vi "ref Periodic Tasks.vi"(8 "error in":errorcluster) -> ()   [LabVIEW 2020]
doc: "This VI runs in parallel to other tasks. It can contain as many user-defined periodic loops as you need. These can carry out PID or other sorts of timed response."
uses:
  <vilib>/Rock Robotics/Network Tables/NT Write Number.vi
  <vilib>/Rock Robotics/Network Tables/NT Write String.vi
  <vilib>/Rock Robotics/WPI/ThirdParty/Sensors/navX/_TypeDefs/FRIC_navX_DeviceNumbersTypeDef.ctl
  <vilib>/Rock Robotics/SystemInterfaces/i2clib/i2c_bus.ctl
  <vilib>/Rock Robotics/WPI/ThirdParty/Sensors/navX/_Processing Loop/FRIC_navX_Internal_I2C_ProcessingLoop.vi
  <vilib>/Rock Robotics/Network Tables/NT Read Number.vi
  <vilib>/Rock Robotics/WPI/Ultrasonic/WPI_SonarSRF04DigitalGetRange.vi
  <vilib>/Rock Robotics/WPI/Ultrasonic/WPI_SonarSRF04DigitalRefNum Registry Get.vi
  <vilib>/Rock Robotics/WPI/Ultrasonic/WPI_UltrasonicRangeUnits.ctl
  <vilib>/Rock Robotics/SystemInterfaces/DIO/FPGA_DIOPWMChannel.ctl
  <vilib>/Rock Robotics/WPI/PWM/WPI_PWMDeadband.ctl
  <vilib>/Rock Robotics/WPI/PWM/Servo/WPI_ServoDeviceRef.ctl
panel:
  in  "SONAR ref names":string[](array[string])=["BALL1", "BALL2"]
  in  "Cluster":T4={"RefAngle"="", "RefSetAngle"="", "ServoDeviceRef"={"DeviceStatus"={"status"=FALSE, "code"=0, "source"=""}, "PWM Channel"=enum."Invalid", "DeadBand"={"Name"="", "maxPositivePwm"=0, "minPositivePwm"=0, "centerPwm"=0, "maxNegativePwm"=0, "minNegativePwm"=0, "angularRange"=0}}}
  in  "list of NEO RefNum":string[](array[string])=["ARMLEFT", "ARMRIGHT"]
  in  "list of Falcon 500 RefNum":string[](array[string])=["DriveLEFT", "DriveRIGHT", "ClimberLEFT", "ClimberRIGHT", "SHOOTER"]
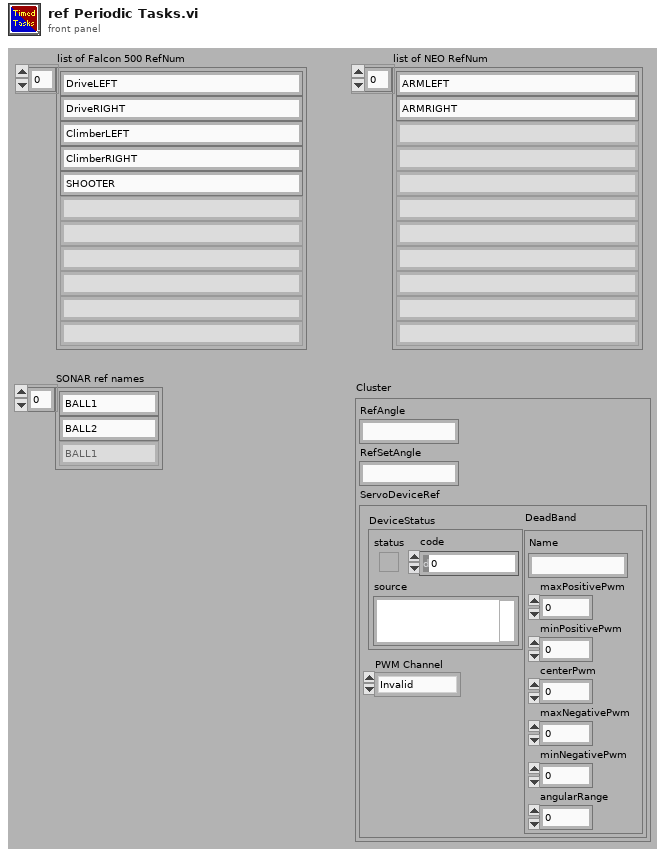
[diagram p1: front panel]
types:
  T1 = typedef "WPI_ServoDeviceRef.ctl" = cluster{"DeviceStatus":errorcluster, "PWM Channel":T2, "DeadBand":T3}
  T2 = typedef "FPGA_DIOPWMChannel.ctl" = enum8{"PWM 0", "PWM 1", "PWM 2", "PWM 3", "PWM 4", "PWM 5", "PWM 6", "PWM 7", "PWM 8", "PWM 9", "PWM MXP 0", "PWM MXP 1", "PWM MXP 2", "PWM MXP 3", "PWM MXP 4", "PWM MXP 5", "PWM MXP 6", "PWM MXP 7", "PWM MXP 8", "PWM MXP 9", "Invalid"}
  T3 = typedef "WPI_PWMDeadband.ctl" = cluster{"Name":string, "maxPositivePwm":i32, "minPositivePwm":i32, "centerPwm":i32, "maxNegativePwm":i32, "minNegativePwm":i32, "angularRange":u16}
  T4 = cluster{"RefAngle":string, "RefSetAngle":string, "ServoDeviceRef":T1}
  T5 = cluster{"RefAngle":string, "RefSetAngle":string, "ServoDeviceRef":T1}[]
  T6 = typedef "i2c_bus.ctl" = enum16{"I2C On-Board", "I2C MXP", "Invalid"}
  T7 = typedef "FRIC_navX_DeviceNumbersTypeDef.ctl" = enum16{"Dev0", "Dev1", "Dev2", "Dev3"}
  T8 = typedef "WPI_UltrasonicDeviceRef.ctl" = cluster{"DevStatus":errorcluster, "Ping Channel":T9, "Echo Channel":T9, "CntIndex":T10}
  T9 = typedef "FPGA_DIOChannel.ctl" = enum8{"DIO 0", "DIO 1", "DIO 2", "DIO 3", "DIO 4", "DIO 5", "DIO 6", "DIO 7", "DIO 8", "DIO 9", "DIO MXP 0", "DIO MXP 1", "DIO MXP 2", "DIO MXP 3", "DIO MXP 4", "DIO MXP 5", "DIO MXP 6", "DIO MXP 7", "DIO MXP 8", "DIO MXP 9", "DIO MXP 10", "DIO MXP 11", "DIO MXP 12", "DIO MXP 13", "DIO MXP 14", "DIO MXP 15", "SPI Port CS1", "SPI Port CS2", "SPI Port CS3", "SPI Port MISO", "SPI Port MOSI", "Invalid"}
  T10 = typedef "FPGA_CounterCtrSystemIndex.ctl" = enum8{"Ctr 0", "Ctr 1", "Ctr 2", "Ctr 3", "Ctr 4", "Ctr 5", "Ctr 6", "Ctr 7", "Invalid"}
  T11 = typedef "WPI_JoystickDevRef.ctl" = cluster{"Device":T12}
  T12 = typedef "WPI_JoystickDeviceEnum.ctl" = enum16{"USB 0", "USB 1", "USB 2", "USB 3", "USB 4", "USB 5"}
  T13 = typedef "WPI_RobotDriveDevRef.ctl" = cluster{"DevStatus":errorcluster, "Motors[]":T14[], "Square Inputs":bool, "Max Output":dbl}
  T14 = typedef "WPI_MotorControlDeviceRef.ctl" = cluster{"DeviceStatus":errorcluster, "Type":T15, "PWM":cluster{"PWM Channel":T2, "DeadBand":T3}, "CAN":cluster{"Device Number":u8, "SetOutput VI Ref":variant, "GetOutput VI Ref":variant, "Enable VI Ref":variant, "Disable VI Ref":variant, "Data":variant}, "Invert":bool, "DIO PWM":cluster{"PWM \"Enable\" Channel":T2, "DIOChannel":T9, "PWM Rate":dbl}}
  T15 = typedef "WPI_MotorControlType.ctl" = enum16{"PWM", "CAN", "DIO PWM"}
  T16 = cluster{"JoystickDevRef":T11, "RobotDriveDevRef":T13}
  T17 = typedef "WPI_UltrasonicRangeUnits.ctl" = enum16{"inches", "mm"}
  T18 = typedef "WPI_DriverStationPositionInfo.ctl" = enum16{"1", "2", "3"}
  T19 = typedef "WPI_DriverStationAllianceInfo.ctl" = enum16{"Red", "Blue", "Invalid"}
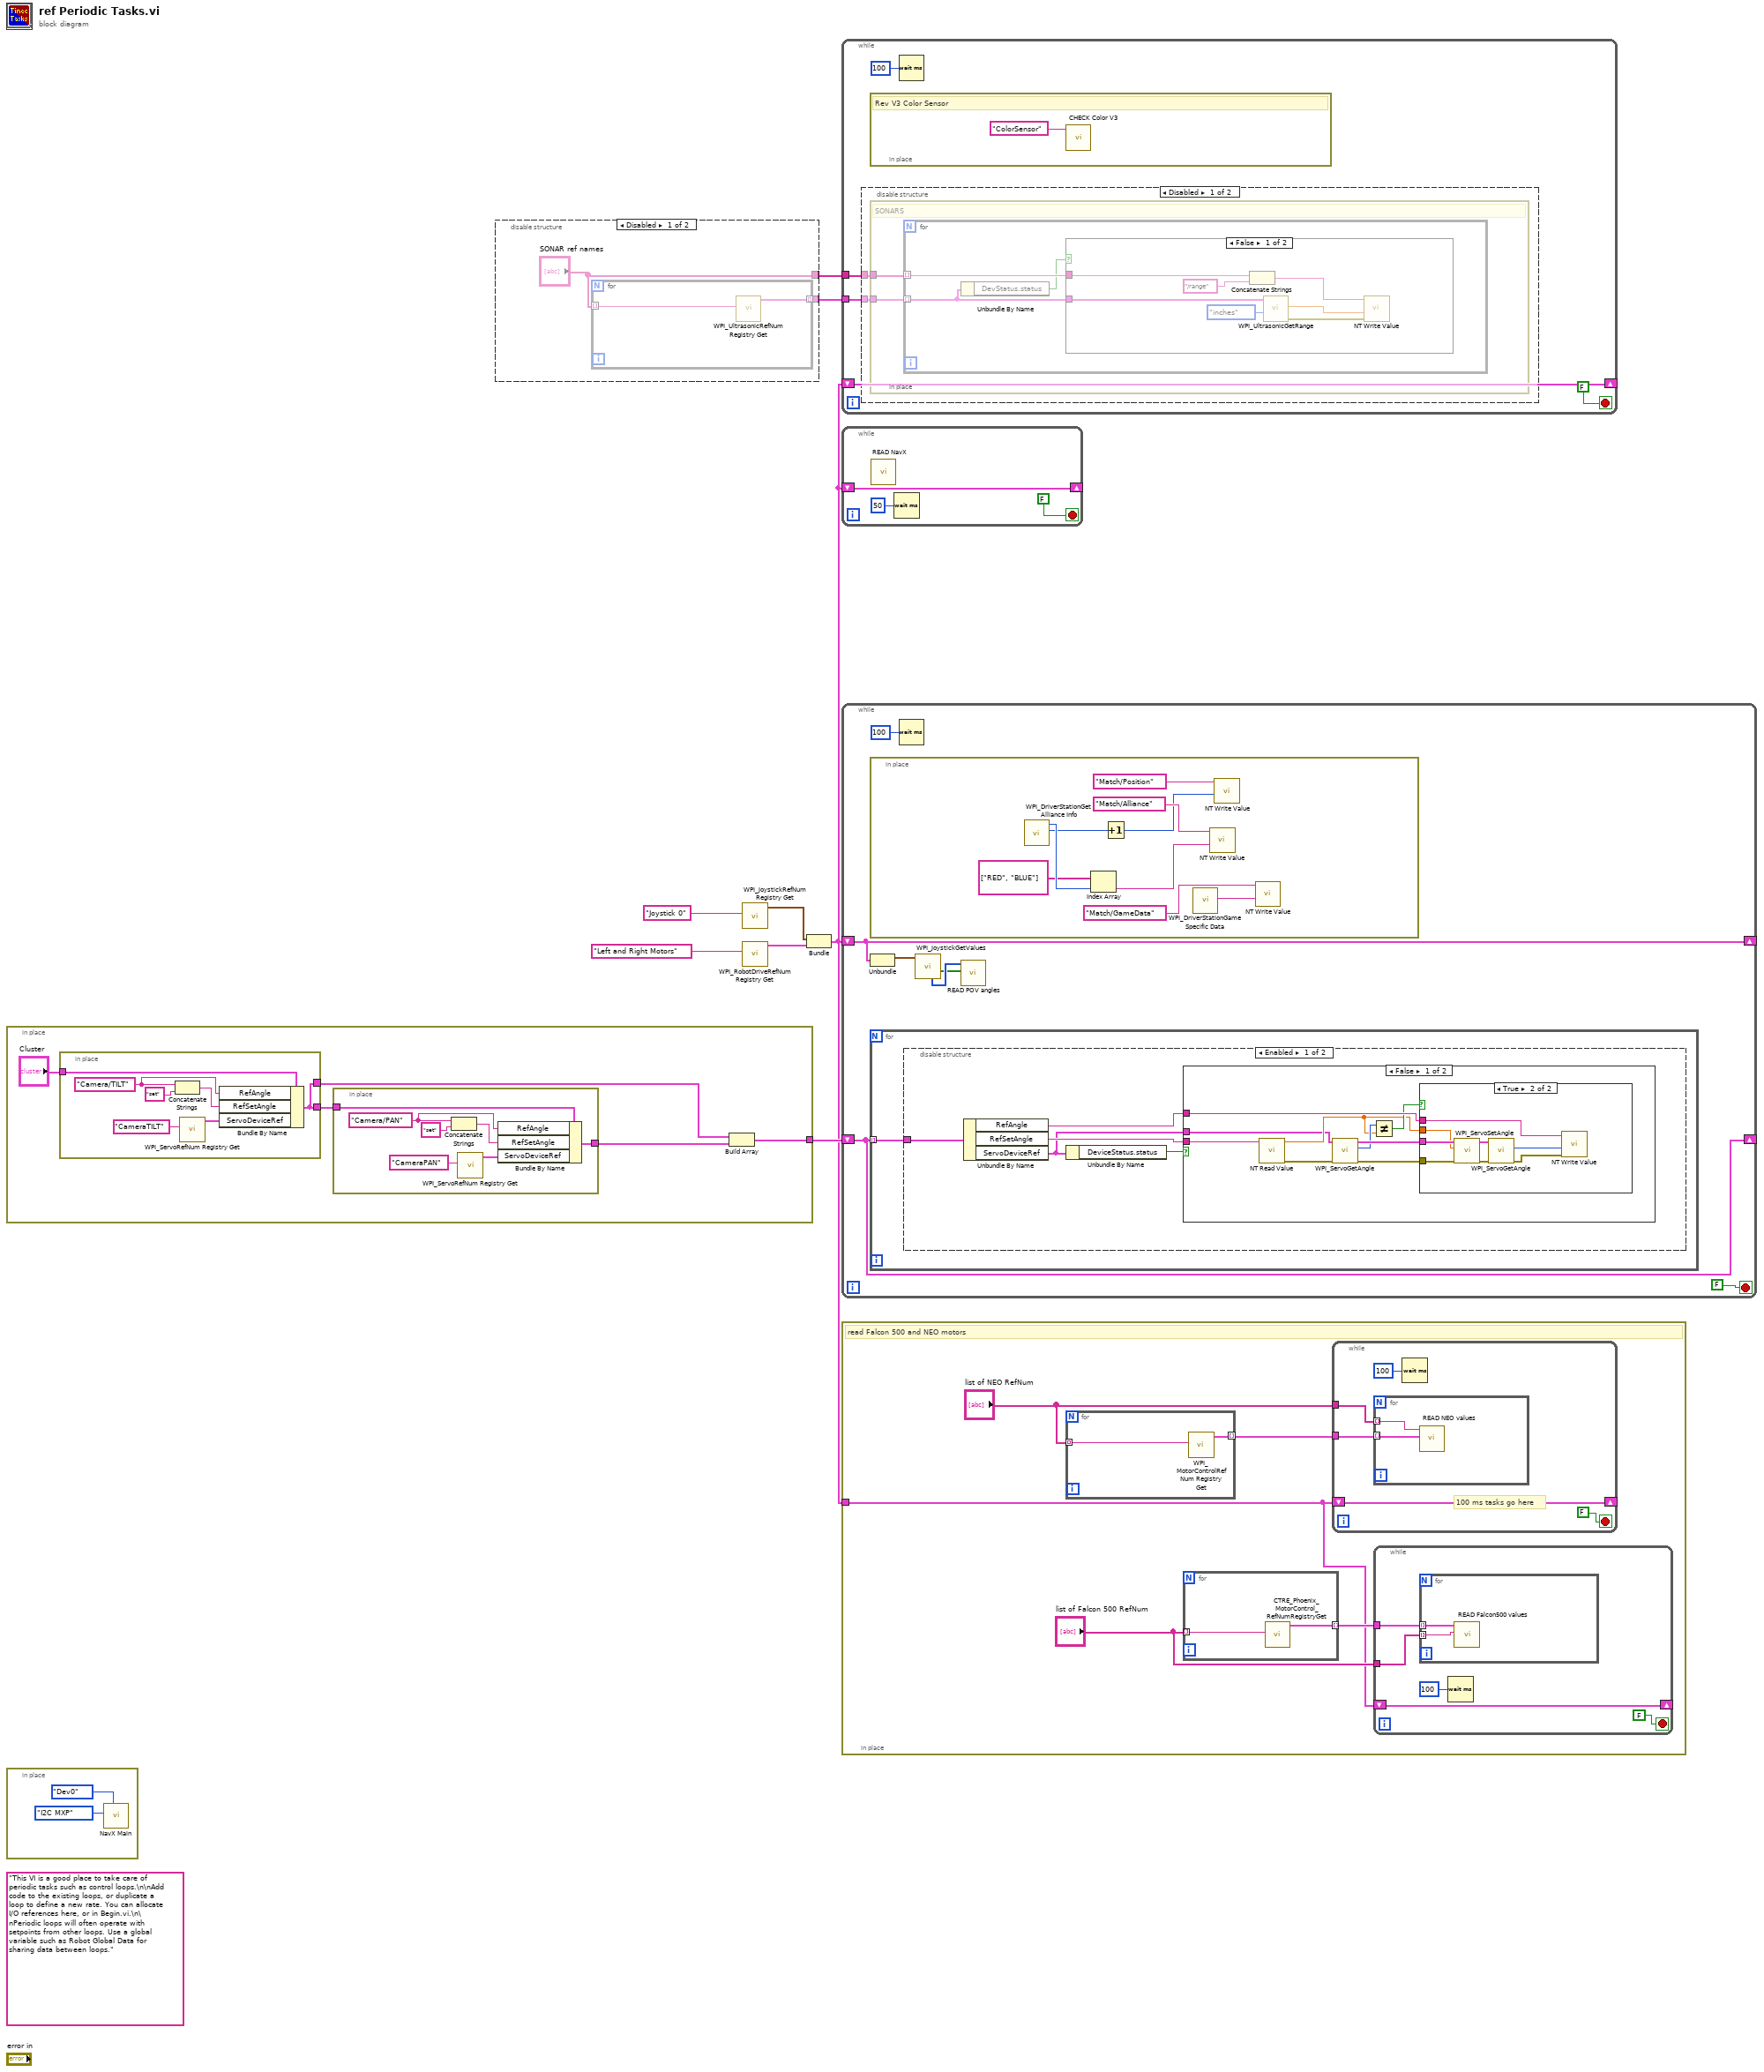
[diagram p0: block diagram]
diagram:
  (unwired) "This VI is a good place to take care of periodic tasks such as control loops.\n\nAdd code to the existing loops, or duplicate a loop to define a new rate. You can allocate I/O references here, or in Begin.vi.\n\nPeriodic loops will often operate with setpoints from other loops. Use a global variable such as Robot Global Data for sharing data between loops."
  n1 = in-place {
    in-place-border: [w11] -> w4
    n2 = in-place {
      in-place-border: "Cluster" -> [w27]
      in-place-border: [w23] -> w13
      in-place-border: [w23] -> w10
      w25 = "Camera/TILT" ("Name")
      n3 = Concatenate Strings(w25, "set" ("string")) -> (w26:string)
      n4 = call <vilib>:"WPI_ServoRefNum Registry Get.vi"("refnum name"="CameraTILT") -> ("ServoDeviceRef"=w21:T1)  [unwired: 9 in, 1 out]
      n5 = Bundle By Name(cluster=w27, "RefAngle"=w25, "RefSetAngle"=w26, "ServoDeviceRef"=w21) -> (w23:T4)
    }
    n6 = in-place {
      in-place-border: [w17] -> w12
      in-place-border: w10 -> [w16]
      w19 = "Camera/PAN" ("Name")
      n7 = Concatenate Strings(w19, "set" ("string")) -> (w20:string)
      n8 = call <vilib>:"WPI_ServoRefNum Registry Get.vi"("refnum name"="CameraPAN") -> ("ServoDeviceRef"=w14:T1)  [unwired: 9 in, 1 out]
      n9 = Bundle By Name(cluster=w16, "RefAngle"=w19, "RefSetAngle"=w20, "ServoDeviceRef"=w14) -> (w17:T4)
    }
    n10 = Build Array(w13, w12) -> (w11:T5)
  }
  n11 = in-place {
    n12 = call-poly <vilib>:"NavX Main.vi"("Device Number"=FRIC_navX_DeviceNumbersTypeDef."Dev0", "I2C Bus"=i2c_bus."I2C MXP") -> ()  [unwired: 10 in]
  }
  n13 = disable-structure shown="Disabled" {
    disable-tunnel: ["SONAR ref names" _] -> w2
    disable-tunnel: [w30 _] -> w1
    frame Disabled {
      n14 = for {
        tunnel: "SONAR ref names" -> [w33] mode=indexing
        tunnel: [w32] -> w30 mode=indexing
        n15 = call-poly <vilib>:"WPI_UltrasonicRefNum Registry Get.vi"("refnum name"=w33) -> ("SonarSRF04DevRef"=w32:T8)  [unwired: 9 in, 1 out]
      }
    }
    frame Enabled {
    }
  }
  n16 = call <vilib>:"WPI_JoystickRefNum Registry Get.vi"("refnum name"="Joystick 0") -> ("JoystickDevRef"=w6:T11)  [unwired: 1 in, 9 out]
  n17 = call <vilib>:"WPI_RobotDriveRefNum Registry Get.vi"("refnum name"="Left and Right Motors") -> ("RobotDriveDevRef"=w5:T13)  [unwired: 1 in, 9 out]
  n18 = Bundle("JoystickDevRef"=w6, "RobotDriveDevRef"=w5) -> (w3:T16)  [unwired: 1 out]
  n19 = while {
    shift-right: [w34] -> _
    shift-left: w3 -> [w34]
    tunnel: w2 -> [w36]
    tunnel: w1 -> [w35]
    stop <- FALSE stop-if-true
    n20 = disable-structure shown="Disabled" {
      disable-tunnel: w36 -> [w40 _]
      disable-tunnel: w35 -> [w39 _]
      frame Disabled {
        n21 = in-place {
          in-place-border: w40 -> [w42]
          in-place-border: w39 -> [w41]
          # "SONARS"
          n22 = for {
            tunnel: w42 -> [w45] mode=indexing
            tunnel: w41 -> [w43] mode=indexing
            n23 = Unbundle By Name(w43) -> ("DevStatus.status"=w44:bool)
            n24 = case shown="False" w44 {
              tunnel: w45 -> [w48 _]
              tunnel: w43 -> [w47 _]
              frame False {
                n25 = Concatenate Strings(w48, "/range" ("string")) -> (w52:string)
                n26 = call-poly <vilib>:"WPI_UltrasonicGetRange.vi"("Range Units"=WPI_UltrasonicRangeUnits."inches", "UltrasonicDevRef"=w47) -> ("error out"=w50:errorcluster, "Distance"=w49:dbl)  [unwired: 7 in, 1 out]
                n27 = call-poly <vilib>:"NT Write Value.vi"("error in"=w50, "Numeric"=w49, "Name"=w52) -> ()  [unwired: 8 in, 1 out]
              }
              frame True {
              }
            }
          }
        }
      }
      frame Enabled {
      }
    }
    n28 = in-place "In Place Element Structure" {
      # "Rev V3 Color Sensor"
      n29 = call "CHECK Color V3.vi"("refnum name"="ColorSensor") -> ()  [unwired: 6 in, 5 out]
    }
    n30 = Wait (ms)(milliseconds to wait=u32 100) -> ()  [unwired: 1 out]
  }
  n31 = while {
    shift-right: [w55] -> _
    shift-left: w3 -> [w55]
    stop <- FALSE stop-if-true
    n32 = call "READ NavX.vi"() -> ()  [unwired: 12 in]
    n33 = Wait (ms)(milliseconds to wait=u32 50) -> ()  [unwired: 1 out]
  }
  n34 = while {
    shift-right: [w60] -> _
    shift-left: w3 -> [w60]
    shift-right: [w61] -> _
    shift-left: w4 -> [w61]
    stop <- FALSE stop-if-true
    n35 = in-place {
      n36 = call <vilib>:"WPI_DriverStationGet Alliance Info.vi"() -> ("Position"=w92:T18, "Alliance"=w95:T19)  [unwired: 6 in, 4 out]
      n37 = Index Array(array=string[] ["RED", "BLUE"], index=w95) -> (element=w89:string)
      n38 = Increment(x=w92) -> (x+1=w87:T18)
      n39 = call <vilib>:"WPI_DriverStationGame Specific Data.vi"() -> ("Game Specific Data"=w90:string)  [unwired: 11 in]
      n40 = call-poly <vilib>:"NT Write Value.vi"("String"=w89, "Name"="Match/Alliance") -> ()  [unwired: 9 in, 1 out]
      n41 = call-poly <vilib>:"NT Write Value.vi"("Numeric"=w87, "Name"="Match/Position") -> ()  [unwired: 9 in, 1 out]
      n42 = call-poly <vilib>:"NT Write Value.vi"("String"=w90, "Name"="Match/GameData") -> ()  [unwired: 9 in, 1 out]
    }
    n43 = Unbundle(w60) -> ("JoystickDevRef"=w59:T11)  [unwired: 1 out]
    n44 = for {
      tunnel: w61 -> [w64] mode=indexing
      n45 = disable-structure shown="Enabled" {
        disable-tunnel: w64 -> [w67 _]
        frame Enabled {
          n46 = Unbundle By Name(w67) -> ("RefAngle"=w68:string, "RefSetAngle"=w69:string, "ServoDeviceRef"=w66:T1)
          n47 = Unbundle By Name(w66) -> ("DeviceStatus.status"=w65:bool)
          n48 = case shown="False" w65 {
            tunnel: w69 -> [w75 _]
            tunnel: w68 -> [w74 _]
            tunnel: w66 -> [w71 _]
            frame False {
              n49 = call-poly <vilib>:"NT Read Value.vi"("Name"=w75) -> ("error out"=w70:errorcluster, "Numeric"=w72:dbl)  [unwired: 9 in]
              n50 = call <vilib>:"WPI_ServoGetAngle.vi"("ServoDeviceRef"=w71, "error in (no error)"=w70) -> ("ServoDeviceRef"=w77:T1, "Angle"=w76:u16, "error out"=w78:errorcluster)  [unwired: 6 in]
              n51 = Not Equal?(x=w76, y=w72) -> (x != y?=w73:bool)
              n52 = case shown="True" w73 {
                tunnel: w78 -> [_ w86]
                tunnel: w77 -> [_ w85]
                tunnel: w74 -> [_ w84]
                tunnel: w72 -> [_ w83]
                frame False {
                }
                frame True {
                  n53 = call <vilib>:"WPI_ServoSetAngle.vi"("error in (no error)"=w86, "Angle"=w83, "ServoDeviceRef"=w85) -> ("error out"=w81:errorcluster, "ServoDeviceRef"=w82:T1)  [unwired: 7 in]
                  n54 = call <vilib>:"WPI_ServoGetAngle.vi"("ServoDeviceRef"=w82, "error in (no error)"=w81) -> ("Angle"=w79:u16, "error out"=w80:errorcluster)  [unwired: 6 in, 1 out]
                  n55 = call-poly <vilib>:"NT Write Value.vi"("error in"=w80, "Numeric"=w79, "Name"=w84) -> ()  [unwired: 8 in, 1 out]
                }
              }
            }
            frame True {
            }
          }
        }
        frame Disabled {
        }
      }
    }
    n56 = Wait (ms)(milliseconds to wait=u32 100) -> ()  [unwired: 1 out]
    n57 = call <vilib>:"WPI_JoystickGetValues.vi"("JoystickDevRef"=w59) -> ("Buttons"=w57:bool[], "POVs"=w58:i16[])  [unwired: 6 in, 3 out]
    n58 = call "READ POV angles.vi"("Buttons"=w57, "POVs"=w58) -> ()  [unwired: 10 in]
  }
  n59 = in-place {
    in-place-border: w3 -> [w98]
    # "read Falcon 500 and NEO motors"
    n60 = for {
      tunnel: "list of NEO RefNum" -> [w102] mode=indexing
      tunnel: [w101] -> w96 mode=indexing
      n61 = call <vilib>:"WPI_MotorControlRefNum Registry Get.vi"("refnum name"=w102) -> ("MotorControlDevRef"=w101:T14)  [unwired: 9 in, 1 out]
    }
    n62 = for {
      tunnel: "list of Falcon 500 RefNum" -> [w111] mode=indexing
      tunnel: [w110] -> w100 mode=indexing
      n63 = call <vilib>:"CTRE_Phoenix_MotorControl_RefNumRegistryGet.vi"("refnum name"=w111) -> ("PhoenixMotorControlDevRef"=w110:T14)  [unwired: 9 in, 1 out]
    }
    n64 = while {
      shift-right: [w105] -> _
      shift-left: w98 -> [w105]
      tunnel: w96 -> [w104]
      tunnel: "list of NEO RefNum" -> [w103]
      stop <- FALSE stop-if-true
      # "100 ms tasks go here"
      n65 = for {
        tunnel: w104 -> [w109] mode=indexing
        tunnel: w103 -> [w108] mode=indexing
        n66 = call "READ NEO values.vi"("MotorControlDevRef"=w109, "RefName"=w108) -> ()  [unwired: 9 in, 1 out]
      }
      n67 = Wait (ms)(milliseconds to wait=u32 100) -> ()  [unwired: 1 out]
    }
    n68 = while {
      shift-right: [w114] -> _
      shift-left: w98 -> [w114]
      tunnel: w100 -> [w113]
      tunnel: "list of Falcon 500 RefNum" -> [w112]
      stop <- FALSE stop-if-true
      n69 = for {
        tunnel: w113 -> [w118] mode=indexing
        tunnel: w112 -> [w117] mode=indexing
        n70 = call "READ Falcon500 values.vi"("PhoenixMotorControlDevRef"=w118, "refnum name"=w117) -> ()  [unwired: 6 in, 2 out]
      }
      n71 = Wait (ms)(milliseconds to wait=u32 100) -> ()  [unwired: 1 out]
    }
  }
